vi "Control de reles.vi"() -> ()   [LabVIEW 2019]
panel:
  in  "Control de Caragas":T1(ring)
  in  "Stop":bool=TRUE
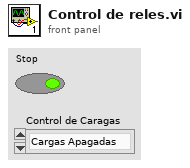
[diagram p1: front panel]
types:
  T1 = enum16{"Cargas Apagadas", "Activar Primer Carga", "Activar Segunda Carga", "Activar Ambas Cargas"}
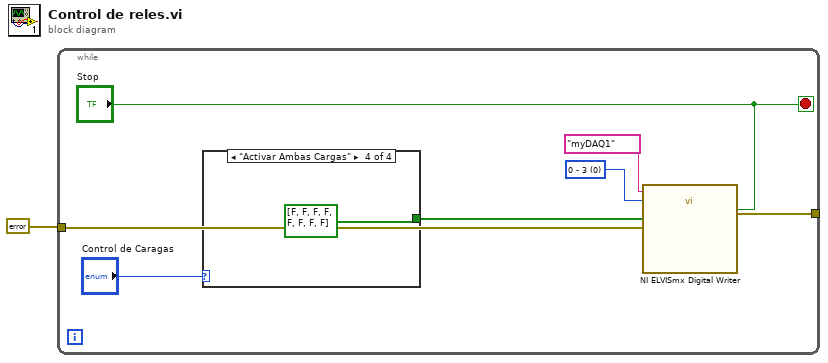
[diagram p0: block diagram]
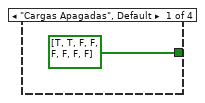
[diagram p2: hidden frame]
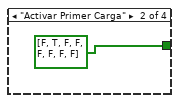
[diagram p3: hidden frame]
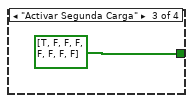
[diagram p4: hidden frame]
diagram:
  n1 = while {
    tunnel: errorcluster {"status"=FALSE, "code"=0, "source"=""} ("error in") -> [w5]
    tunnel: [w2] -> _
    stop <- "Stop" stop-if-true
    w6 = u16 0 items=["0 - 3", "4 - 7", "0 - 7"] ("myDAQ Lines to Write")
    n2 = case shown="\"Activar Ambas Cargas\"" "Control de Caragas" {
      tunnel: [bool[] [TRUE, TRUE, FALSE, FALSE, FALSE, FALSE, FALSE, FALSE] ("DO Lines") bool[] [FALSE, TRUE, FALSE, FALSE, FALSE, FALSE, FALSE, FALSE] ("DO Lines") bool[] [TRUE, FALSE, FALSE, FALSE, FALSE, FALSE, FALSE, FALSE] ("DO Lines") bool[] [FALSE, FALSE, FALSE, FALSE, FALSE, FALSE, FALSE, FALSE] ("DO Lines")] -> w4
      frame "Cargas Apagadas", Default {
      }
      frame "Activar Primer Carga" {
      }
      frame "Activar Segunda Carga" {
      }
      frame "Activar Ambas Cargas" {
      }
    }
    n3 = call "NI ELVISmx Digital Writer"("Device Name"=tag "myDAQ1", "myDAQ Lines to Write"=w6, "Stop"="Stop", "DO Lines"=w4, "error in"=w5) -> ("error out"=w2:errorcluster)  [unwired: 14 in]
  }
